vi "Daq devices.vi"(7 "error in":errorcluster) -> (0 "error out":errorcluster, 1 "AO":string, 2 "AI":string, 3 "DO":string, 4 "Devices":string[](array[string]))   [LabVIEW 2012]
uses:
  <vilib>/nisyscfg/nisyscfg.lvlib
  <resource>/objmgr/nisysapi.rc
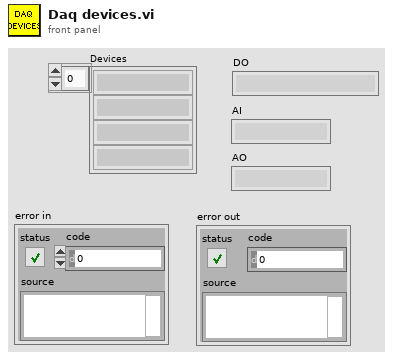
[diagram p1: front panel]
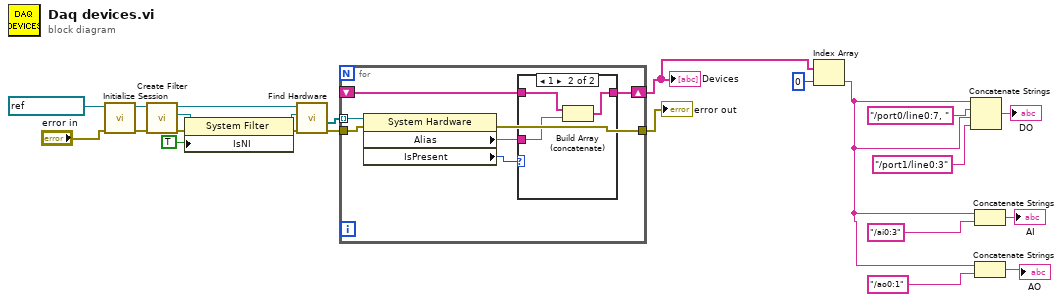
[diagram p0: block diagram]
diagram:
  n1 = call <vilib>:"Initialize Session.vi"("error in (no error)"="error in", "target (localhost)"=refnum<k21> "localhost" ("Target (localhost)")) -> ("error out"=w18:errorcluster, "session out"=w19:refnum<k21>)  [unwired: 8 in]
  n2 = call <vilib>:"Create Filter.vi"("error in (no error)"=w18, "session in"=w19) -> ("error out"=w14:errorcluster, "filter out"=w17:refnum<k20>, "session out"=w20:refnum<k21>)  [unwired: 7 in]
  n3 = property class="System Filter"(reference=w17, error in=w14, "IsNI"=TRUE ("Is Device")) -> (reference out=w16:refnum<k20>, error out=w13:errorcluster)
  n4 = call <vilib>:"Find Hardware.vi"("error in (no error)"=w13, "filter in"=w16, "session in"=w20) -> ("error out"=w22:errorcluster, "resources out"=w12:refnum<k20>[])  [unwired: 1 in, 6 out]
  n5 = for {
    tunnel: w12 -> [w30] mode=indexing
    tunnel: [w29] -> w23
    tunnel: w22 -> [w28]
    shift-right: [w24] -> w7
    shift-left: _ -> [w25]
    n6 = property class="System Hardware"(reference=w30, error in=w28) -> (error out=w29:errorcluster, "Alias"=w26:string, "IsPresent"=w27:i32)  [unwired: 1 out]
    n7 = case shown="1" w27 {
      tunnel: w26 -> [_ w34]
      tunnel: w25 -> [w31 w33]
      tunnel: [w31 w32] -> w24
      frame 0, Default {
      }
      frame 1 {
        n8 = Build Array (concatenate)(w33, w34) -> (w32:string[])
      }
    }
  }
  "error out" <- w23
  "Devices" <- w7
  n9 = Index Array(array=w7, index=0) -> (element=w3:string)
  n10 = Concatenate Strings(w3, "/port0/line0:7, ", w3, "/port1/line0:3") -> (→"DO":string)
  n11 = Concatenate Strings(w3, "/ai0:3") -> (→"AI":string)
  n12 = Concatenate Strings(w3, "/ao0:1") -> (→"AO":string)
